vi "Wrapper_openAllSpectrometers_Mod.vi"(8 "error in (no error)":errorcluster caption="entrée d'erreur (pas d'erreur)", 10 "Wrapper In":u32) -> (0 "error out":errorcluster caption="sortie d'erreur", 2 "Wrapper Out":u32, 3 "Number of Spectrometers":i32)   [LabVIEW 2024]
uses:
  Program Files (x86)/Ocean Optics/OmniDriver/OOI_HOME/OmniDriver32.dll
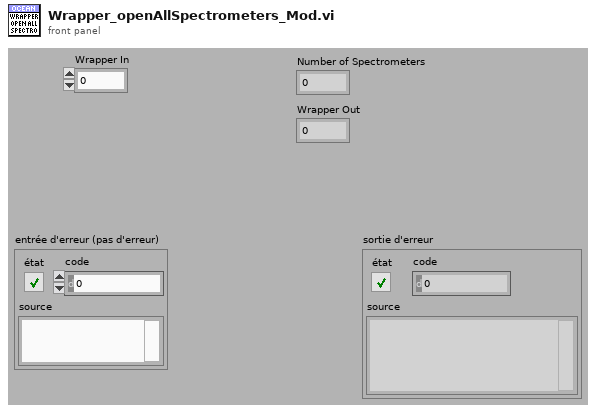
[diagram p1: front panel]
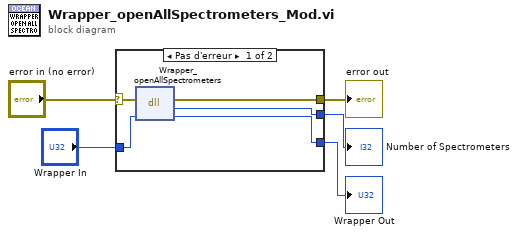
[diagram p0: block diagram]
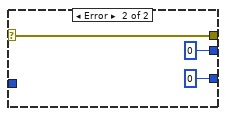
[diagram p2: hidden frame]
diagram:
  n1 = case shown="Pas d'erreur" "error in (no error)" {
    selector: "error in (no error)" -> [w7 w13]
    tunnel: [w10 0 ("Wrapper")] -> w5
    tunnel: [w9 u32 0 ("Wrapper")] -> w4
    tunnel: "Wrapper In" -> [w8 _]
    tunnel: [w6 w13] -> w1
    frame No Error {
      n2 = dll-call lib="C:/Program Files (x86)/Ocean Optics/OmniDriver/OOI_HOME/OmniDriver32.dll" fn="Wrapper_openAllSpectrometers" label="Wrapper.openAllSpectrometers"(error in=w7, "Wrapper"=w8) -> (error out=w6:errorcluster, w10:i32, "Wrapper"=w9:u32)  [unwired: 2 in, 1 out]
    }
    frame Error {
    }
  }
  "Number of Spectrometers" <- w5
  "Wrapper Out" <- w4
  "error out" <- w1
